vi "data_savetxt.vi"(7 "Save":bool, 8 "error in (no error)":errorcluster, 11 "ParasOutput":string) -> (0 "error out":errorcluster, 3 "path_out":path)   [LabVIEW 2022 SP3]
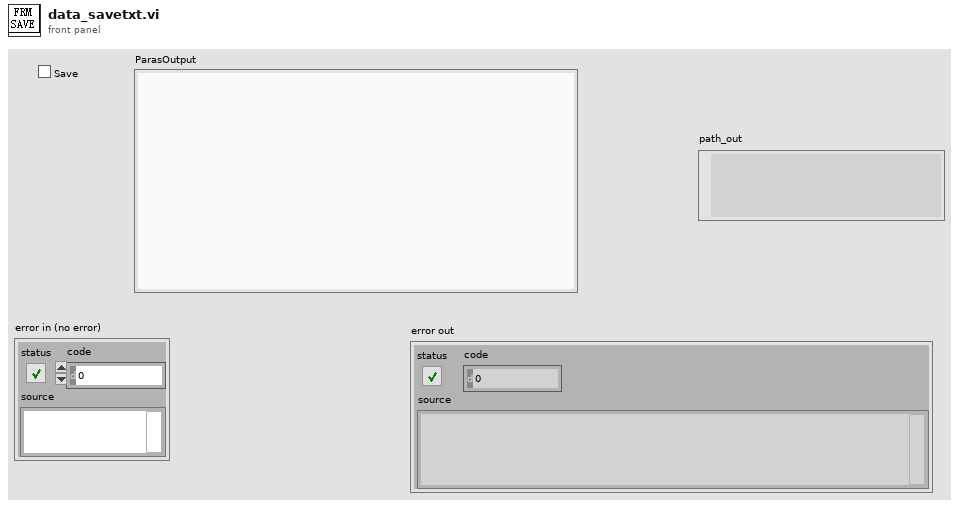
[diagram p1: front panel]
types:
  T1 = enum16{"open", "replace", "create", "open or create", "replace or create", "replace or create with confirmation"}
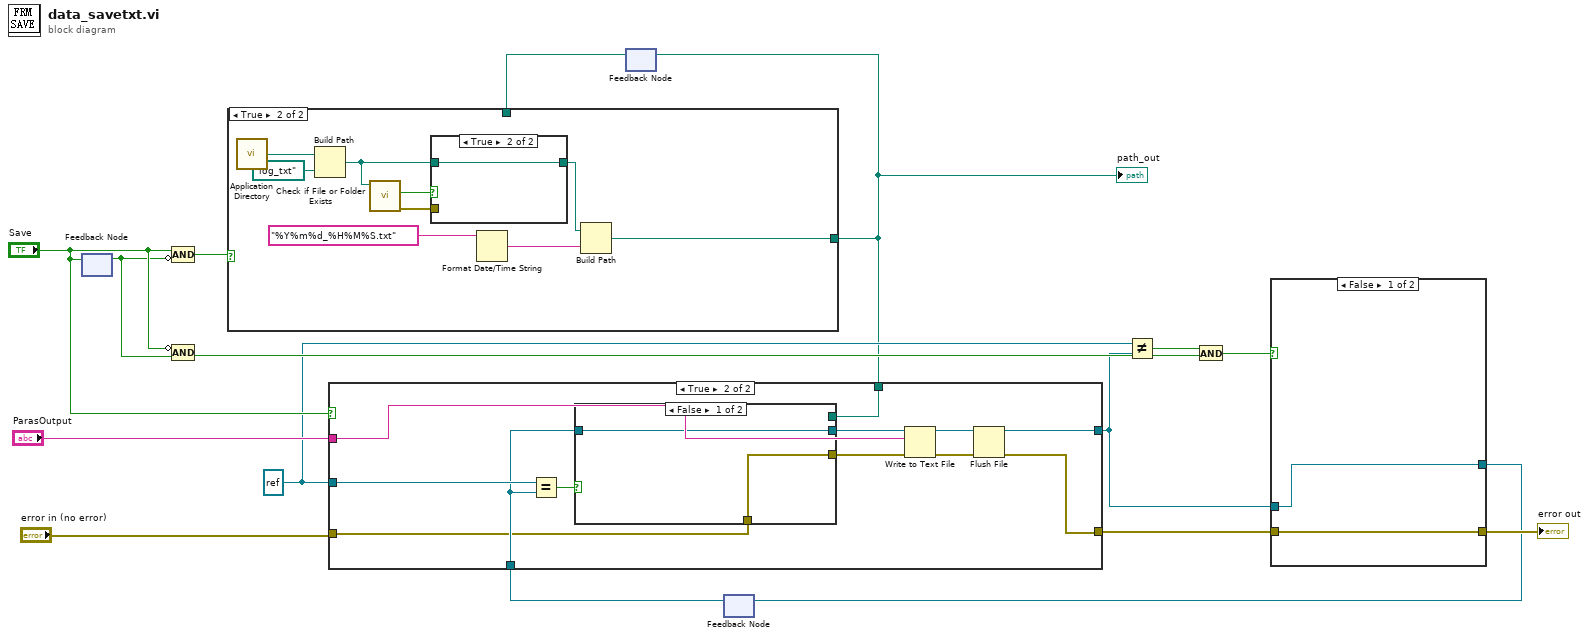
[diagram p0: block diagram]
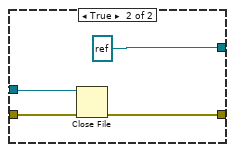
[diagram p2: hidden frame]
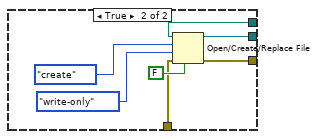
[diagram p4: hidden frame]
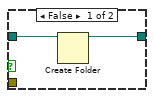
[diagram p6: hidden frame]
diagram:
  w3 = refnum<file> refnum ("refnum out")
  n1 = feedback-in #1("Save") -> ()
  n2 = feedback #1() -> (w11:bool)  [unwired: 1 in]
  n3 = Compound Arithmetic op=AND("Save", invert w11) -> (w13:bool)
  n4 = Compound Arithmetic op=AND(invert "Save", w11) -> (w9:bool)
  n5 = feedback #2() -> (w16:path)  [unwired: 1 in]
  n6 = case shown="True" w13 {
    tunnel: [w17 w18] -> w1
    tunnel: w16 -> [w17 _]
    frame False {
    }
    frame True {
      n7 = call <vilib>:"Application Directory.vi"() -> ("Application Directory"=w24:path)
      n8 = Build Path(base path=w24, name or relative path=path "log_txt") -> (appended path=w21:path)
      n9 = call <vilib>:"Check if File or Folder Exists.vi"("path"=w21) -> ("error out"=w20:errorcluster, "file or folder exists?"=w22:bool)  [unwired: 8 in, 1 out]
      n10 = case shown="True" w22 {
        tunnel: w21 -> [w28 w29]
        tunnel: w20 -> [_ _]
        tunnel: [w27 w29] -> w19
        frame False {
          n11 = Create Folder(path (use dialog)=w28) -> (created path=w27:path)  [unwired: 2 in, 2 out]
        }
        frame True {
        }
      }
      n12 = Format Date/Time String(time format string (%c)="%Y%m%d_%H%M%S.txt") -> (date/time string=w25:string)  [unwired: 2 in]
      n13 = Build Path(base path=w19, name or relative path=w25) -> (appended path=w18:path)
    }
  }
  "path_out" <- w1
  n14 = feedback-in #2(w1) -> ()
  n15 = feedback #3() -> (w4:refnum<file>)  [unwired: 1 in]
  n16 = case shown="True" "Save" {
    tunnel: w1 -> [_ w34]
    tunnel: "error in (no error)" -> [w31 w32]
    tunnel: [w31 w39] -> w7
    tunnel: "ParasOutput" -> [_ w43]
    tunnel: [w30 w40] -> w5
    tunnel: w4 -> [w30 w35]
    tunnel: w3 -> [_ w36]
    frame False {
    }
    frame True {
      n17 = Equal?(x=w36, y=w35) -> (x = y?=w37:bool)
      n18 = case shown="False" w37 {
        tunnel: [w45 w49] -> w38
        tunnel: w35 -> [w45 _]
        tunnel: w34 -> [_ w48]
        tunnel: [w44 w47] -> w33
        tunnel: w32 -> [w44 w46]
        frame False {
        }
        frame True {
          n19 = Open/Create/Replace File(file path (use dialog)=w48, error in=w46, operation (0:open)=T1."create", access (0:read/write)=enum16{"read/write", "read-only", "write-only"}."write-only", disable buffering (F)=FALSE) -> (refnum out=w49:refnum<file>, error out=w47:errorcluster)  [unwired: 1 in, 1 out]
        }
      }
      n20 = Write to Text File(file (use dialog)=w38, text=w43, error in=w33) -> (refnum out=w42:refnum<file>, error out=w41:errorcluster)  [unwired: 1 in, 1 out]
      n21 = Flush File(refnum=w42, error in=w41) -> (refnum out=w40:refnum<file>, error out=w39:errorcluster)
    }
  }
  n22 = Not Equal?(x=w3, y=w5) -> (x != y?=w10:bool)
  n23 = And(x=w10, y=w9) -> (x .and. y?=w8:bool)
  n24 = case shown="False" w8 {
    tunnel: w5 -> [w53 w58]
    tunnel: w7 -> [w54 w57]
    tunnel: [w54 w56] -> w6
    tunnel: [w53 refnum<file> refnum ("refnum out")] -> w2
    frame False {
    }
    frame True {
      n25 = Close File(refnum=w58, error in=w57) -> (error out=w56:errorcluster)  [unwired: 1 out]
    }
  }
  "error out" <- w6
  n26 = feedback-in #3(w2) -> ()
